vi "Get IO Configuration.vi"(8 "error in (no error)":errorcluster, 10 "IO Type":string, 11 "Refnum in":T1) -> (0 "error out":errorcluster, 3 "output Table":string[][](array[string]))   [LabVIEW 2018]
uses:
  <vilib>/addons/database/Connection.llb/Conn ObjectReference.ctl
  <vilib>/addons/database/NI_Database_API.lvlib
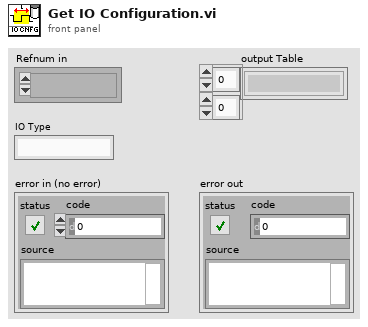
[diagram p1: front panel]
types:
  T1 = typedef "NI_Database_API.lvlib/Conn ObjectReference.ctl" = refnum<k1>
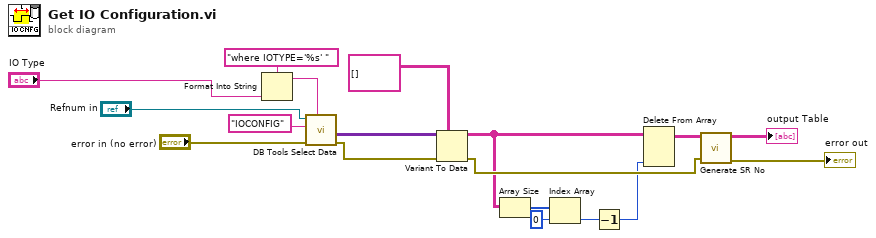
[diagram p0: block diagram]
diagram:
  n1 = Format Into String(format string="where IOTYPE='%s' " ("condition"), "IO Type") -> (resulting string=w16:string)  [unwired: 2 in, 1 out]
  n2 = call <vilib>:"DB Tools Select Data.vi"("condition"=w16, "error in (no error)"="error in (no error)", "table"="IOCONFIG", "connection reference"="Refnum in") -> ("error out"=w12:errorcluster, "data"=w10:variant[][])  [unwired: 2 in, 1 out]
  n3 = Variant To Data(error in=w12, type=string[][] [], Variant=w10) -> (data=w5:string[][], error out=w13:errorcluster)
  n4 = Array Size(array=w5) -> (size(s)=w4:i32[])
  n5 = Index Array(array=w4, index=0) -> (element=w2:i32)
  n6 = Decrement(x=w2) -> (x-1=w1:i32)
  n7 = Delete From Array(array=w5, index (col)=w1) -> (array with subset deleted=w6:string[][])  [unwired: 2 in, 1 out]
  n8 = call "Generate SR No.vi"("error in (no error)"=w13, "Table Control"=w6) -> ("error out"=→"error out":errorcluster, "output Table"=→"output Table":string[][])  [unwired: 8 in]
